vi "Create HHP File.vi"(8 "error in (no error)":errorcluster, 10 "Name of Compiled File":string, 11 "Project Path":path) -> (0 "error out":errorcluster, 2 ".hhp file path":path, 3 "Help Documentation Path":path)   [LabVIEW 2016]
uses:
  Log FGV Operation Modes.ctl
  Error Location.ctl
panel:
  # "(include .chm)"
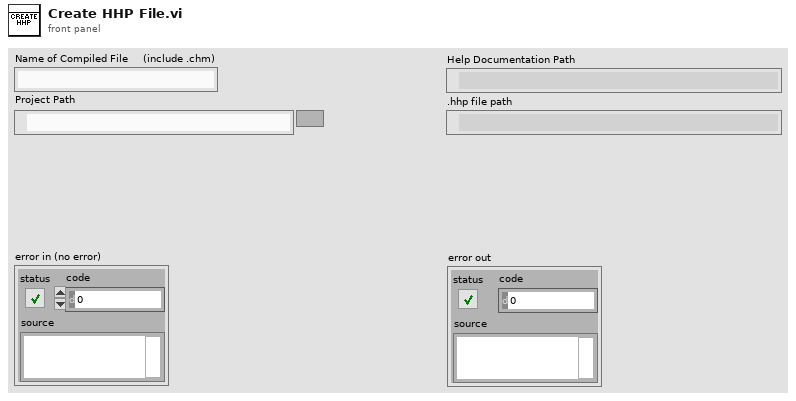
[diagram p1: front panel]
types:
  T1 = typedef "Error Location.ctl" = enum16{"Delete tmp", "Compile HHP", "Find Install", "Create tmp", "Create HHP", "Find Help"}
  T2 = typedef "Log FGV Operation Modes.ctl" = enum16{"Close", "Write", "Open File"}
  T3 = enum16{"open", "replace", "create", "open or create", "replace or create", "replace or create with confirmation"}
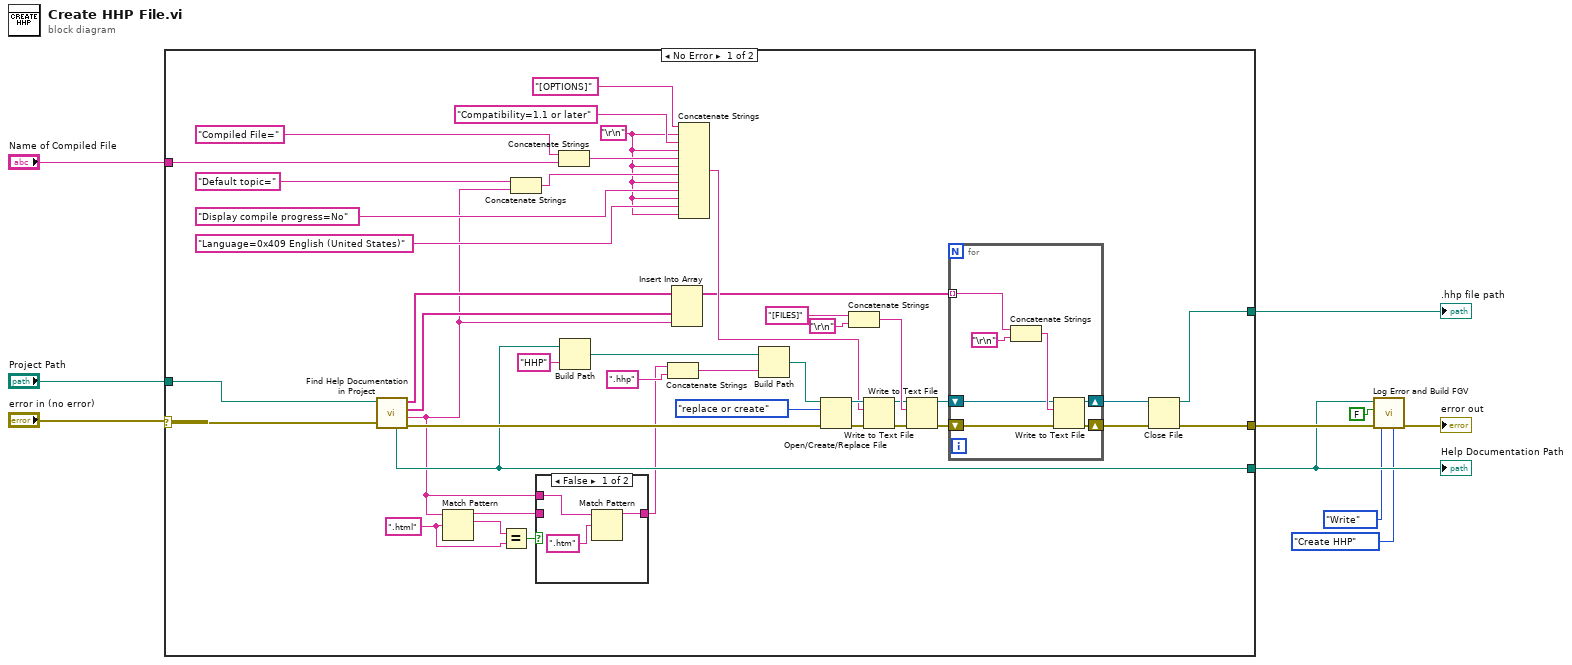
[diagram p0: block diagram]
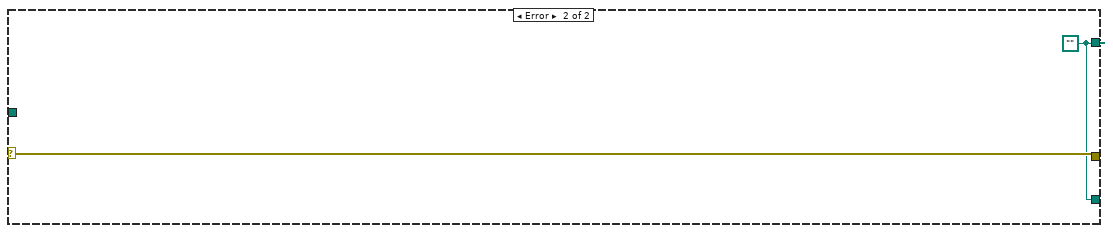
[diagram p3: hidden frame]
diagram:
  n1 = case shown="No Error" "error in (no error)" {
    selector: "error in (no error)" -> [w27 w66]
    tunnel: [w23 w66] -> w6
    tunnel: "Name of Compiled File" -> [w26 _]
    tunnel: "Project Path" -> [w25 _]
    tunnel: [w24 w65] -> w7
    tunnel: [w20 w65] -> w4
    frame No Error {
      w16 = ".html" ("substring (\"\")")
      w28 = "\r\n"
      n2 = call "Find Help Documentation in Project.vi"("error in (no error)"=w27, "Project Path"=w25) -> ("error out"=w49:errorcluster, "Main Page"=w13:string, "Support"=w17:string[], "Other Pages"=w21:string[], "Help Documentation Path"=w20:path)  [unwired: 5 in]
      n3 = Match Pattern(string=w13, regular expression=w16) -> (before substring=w14:string, match substring=w11:string)  [unwired: 1 in, 2 out]
      n4 = Equal?(x=w11, y=w16) -> (x = y?=w15:bool)
      n5 = Concatenate Strings("Default topic=" ("text"), w13) -> (w31:string)
      n6 = case shown="False" w15 {
        tunnel: w14 -> [_ w57]
        tunnel: [w56 w57] -> w12
        tunnel: w13 -> [w55 _]
        frame False {
          n7 = Match Pattern(string=w55, regular expression=".htm") -> (before substring=w56:string)  [unwired: 1 in, 3 out]
        }
        frame True {
        }
      }
      n8 = Concatenate Strings("Compiled File=" ("text"), w26) -> (w32:string)
      n9 = Build Path(base path=w20, name or relative path="HHP") -> (appended path=w18:path)
      n10 = Concatenate Strings(w12, ".hhp" ("string")) -> (w52:string)
      n11 = Insert Into Array(array=w21, new element #1=w17, new element #2=w13) -> (w22:string[])  [unwired: 1 in]
      n12 = Concatenate Strings("[OPTIONS]" ("text"), w28, "Compatibility=1.1 or later" ("text"), w28, w32, w28, w31, w28, "Display compile progress=No" ("text"), w28, "Language=0x409 English (United States)" ("text"), w28) -> (w40:string)
      n13 = Build Path(base path=w18, name or relative path=w52) -> (appended path=w51:path)
      n14 = Open/Create/Replace File(file path (use dialog)=w51, error in=w49, operation (0:open)=T3."replace or create") -> (refnum out=w41:refnum<file>, error out=w37:errorcluster)  [unwired: 3 in, 1 out]
      n15 = Concatenate Strings("[FILES]" ("text"), "\r\n") -> (w42:string)
      n16 = Write to Text File(file (use dialog)=w41, text=w40, error in=w37) -> (refnum out=w38:refnum<file>, error out=w36:errorcluster)  [unwired: 1 in, 1 out]
      n17 = Write to Text File(file (use dialog)=w38, text=w42, error in=w36) -> (refnum out=w47:refnum<file>, error out=w48:errorcluster)  [unwired: 1 in, 1 out]
      n18 = for {
        shift-right: [w60] -> w45
        shift-left: w47 -> [w61]
        shift-right: [w59] -> w46
        shift-left: w48 -> [w64]
        tunnel: w22 -> [w58] mode=indexing
        n19 = Concatenate Strings(w58, "\r\n") -> (w62:string)
        n20 = Write to Text File(file (use dialog)=w61, text=w62, error in=w64) -> (refnum out=w60:refnum<file>, error out=w59:errorcluster)  [unwired: 1 in, 1 out]
      }
      n21 = Close File(refnum=w45, error in=w46) -> (path=w24:path, error out=w23:errorcluster)
    }
    frame Error {
      w65 = path ""
    }
  }
  ".hhp file path" <- w7
  "Help Documentation Path" <- w4
  n22 = call "Log Error and Build FGV.vi"("Error Location"=Error_Location."Create HHP", "Operation Mode"=Log_FGV_Operation_Modes."Write", "error in"=w6, "Log Build Output?"=FALSE, "Help Documentation Path"=w4) -> ("error out"=→"error out":errorcluster)  [unwired: 6 in]
